vi "buildADAMrequest.vi"(9 "Aspect":string(combo), 11 "MFCs":T1[](array[typedef]) {"mDot" format="%_4g"; "Setpoint" format="%.2g"; "MFCcapability"."MaxMdot" format="%_4g"; "MFCcapability"."MinMdot" format="%_4g"}) -> (3 "ADAMrequests":cluster{"String":string, "Setpoint":dbl}[](array[cluster]))   [LabVIEW 2021]
uses:
  MFCdescription.ctl
  MFCcapability.ctl
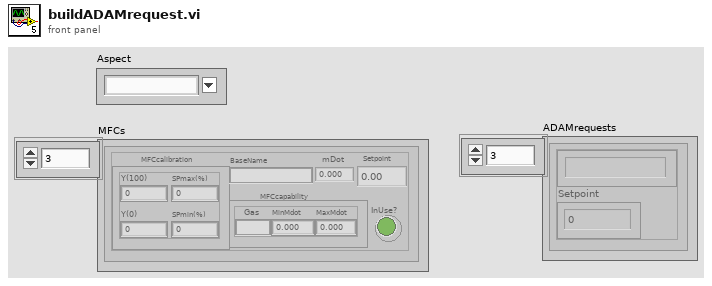
[diagram p1: front panel]
types:
  T1 = typedef "MFCdescription.ctl" = cluster{"BaseName":string, "MFCcalibration":cluster{"Y(100)":dbl, "Y(0)":dbl, "SPmin(%)":dbl, "SPmax(%)":dbl}, "MFCcapability":T2, "InUse?":bool, "Setpoint":dbl, "mDot":dbl}
  T2 = typedef "MFCcapability.ctl" = cluster{"Gas":string, "MinMdot":dbl, "MaxMdot":dbl}
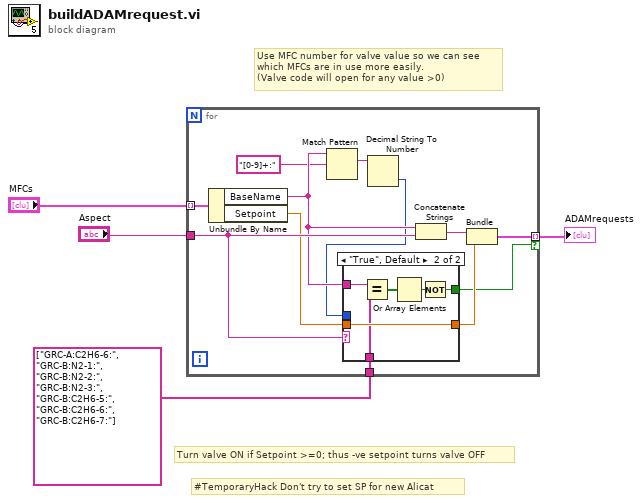
[diagram p0: block diagram]
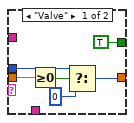
[diagram p2: hidden frame]
diagram:
  # "Use MFC number for valve value so we can see which MFCs are in use more easily.\n(Valve code will open for any value >0)"
  # "#TemporaryHack Don't try to set SP for new Alicat"
  # "Turn valve ON if Setpoint >=0; thus -ve setpoint turns valve OFF"
  n1 = for {
    tunnel: "MFCs" -> [w16] mode=indexing
    tunnel: [w14] -> w4 mode=indexing if=w10
    tunnel: "Aspect" -> [w13]
    tunnel: string[] ["GRC-A:C2H6-6:", "GRC-B:N2-1:", "GRC-B:N2-2:", "GRC-B:N2-3:", "GRC-B:C2H6-5:", "GRC-B:C2H6-6:", "GRC-B:C2H6-7:"] -> [w5]
    n2 = Unbundle By Name(w16) -> ("BaseName"=w9:string, "Setpoint"=w12:dbl)
    n3 = Match Pattern(string=w9, regular expression="[0-9]+:") -> (match substring=w7:string)  [unwired: 1 in, 3 out]
    n4 = Decimal String To Number(string=w7) -> (number=w6:i32)  [unwired: 2 in, 1 out]
    n5 = case shown="\"True\", Default" w13 {
      tunnel: w12 -> [w22 w28]
      tunnel: [w19 w28] -> w11
      tunnel: w9 -> [_ w27]
      tunnel: [TRUE w23] -> w10
      tunnel: w6 -> [w18 _]
      tunnel: w5 -> [_ w25]
      frame "Valve" {
        n6 = Greater Or Equal To 0?(x=w22) -> (x >= 0?=w20:bool)
        n7 = Select(t=w18, s=w20, f=0) -> (s? t:f=w19:i32)
      }
      frame "True", Default {
        n8 = Equal?(x=w27, y=w25) -> (x = y?=w26:bool[])
        n9 = Or Array Elements(Boolean array=w26) -> (logical OR=w24:bool)
        n10 = Not(x=w24) -> (.not. x?=w23:bool)
      }
    }
    n11 = Concatenate Strings(w9, w13) -> (w15:string)
    n12 = Bundle(w15, "Setpoint"=w11) -> (w14:cluster{string, "Setpoint":dbl})  [unwired: 1 in]
  }
  "ADAMrequests" <- w4
